vi "Get Filter Data.vi"(8 "error in (no error)":errorcluster, 11 "Filter XML Ref":refnum<k20>) -> (0 "error out":errorcluster, 1 "Parameters":T1[](array[typedef]) {"Base Word" format="%04d"; "Address" format="%04x"; "Mask" format="%04x"; "Value" format="%016x"}, 2 "Filter Configuration":T3, 3 "Name":string)   [LabVIEW 2016]
doc: "Retrieves all the Bus Monitor Filter Parameters and configuration from the Filter XML node. Each BMChannel should have a unique name. Each Filter should also have a unique name."
uses:
  <vilib>/xml/NI_XML.lvlib
  Frames & Messages/TypeDefs/Command Type.ctl
  BCI-1553 API.lvlib
  Filters/TypeDefs/Filter Configuration.ctl
  1553 SubComponent/TypeDefs/Scaling Information.ctl
  1553 SubComponent/1553 SubComponent.lvclass
  1553 SubComponent/TypeDefs/Parameter Table Data.ctl
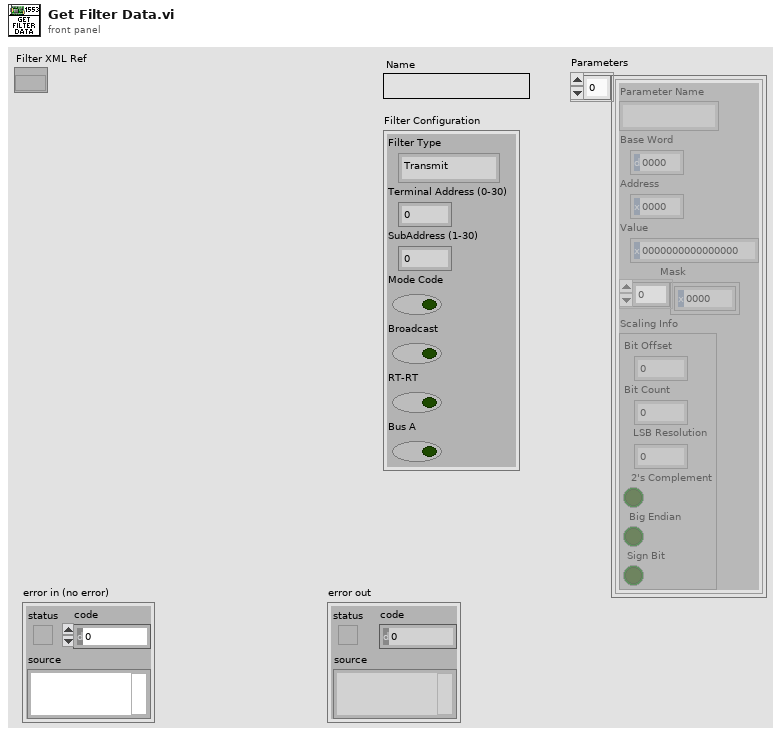
[diagram p1: front panel]
types:
  T1 = typedef "BCI-1553 API.lvlib/1553 SubComponent.lvclass/Parameter Table Data.ctl" = cluster{"Parameter Name":string, "Base Word":u16, "Address":u16, "Value":u64, "Mask":u16[], "Scaling Info":T2}
  T2 = typedef "BCI-1553 API.lvlib/1553 SubComponent.lvclass/Scaling Information.ctl" = cluster{"Bit Offset":i32, "Bit Count":i32, "LSB Resolution":dbl, "2's Complement":bool, "Big Endian":bool, "Sign Bit":bool}
  T3 = typedef "BCI-1553 API.lvlib/Filter Configuration.ctl" = cluster{"Filter Type":T4, "Terminal Address (0-30)":u16, "SubAddress (1-30)":u16, "Mode Code":bool, "Broadcast":bool, "RT-RT":bool, "Bus A":bool}
  T4 = typedef "BCI-1553 API.lvlib/Command Type.ctl" = enum16{"Transmit", "Receive"}
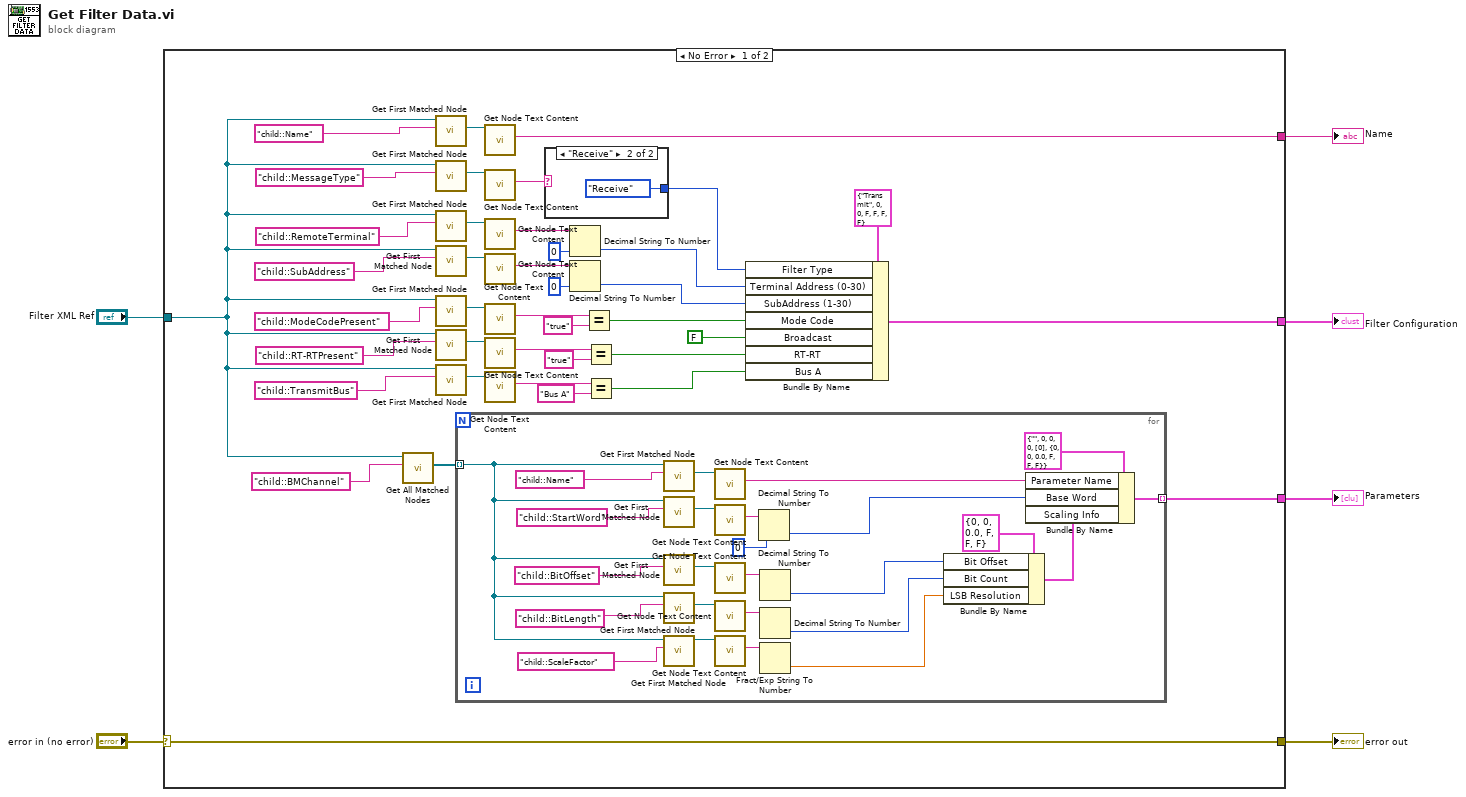
[diagram p0: block diagram]
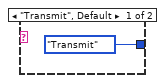
[diagram p2: hidden frame]
diagram:
  n1 = case shown="No Error" "error in (no error)" {
    selector: "error in (no error)" -> [w7 w74]
    tunnel: [w46 _] -> w6
    tunnel: "Filter XML Ref" -> [w45 _]
    tunnel: [w42 _] -> w4
    tunnel: [w41 _] -> w3
    tunnel: [w7 w74] -> w1
    frame No Error {
      n2 = call <vilib>:"Get All Matched Nodes.vi"("XPath expression"="child::BMChannel", "node in"=w45) -> ("node result array"=w40:refnum<k20>[])  [unwired: 7 in, 2 out]
      n3 = call <vilib>:"Get First Matched Node.vi"("XPath expression"="child::Name", "node in"=w45) -> ("node result"=w44:refnum<k20>)  [unwired: 7 in, 2 out]
      n4 = call <vilib>:"Get First Matched Node.vi"("XPath expression"="child::MessageType", "node in"=w45) -> ("node result"=w29:refnum<k20>)  [unwired: 7 in, 2 out]
      n5 = call <vilib>:"Get First Matched Node.vi"("XPath expression"="child::RemoteTerminal", "node in"=w45) -> ("node result"=w23:refnum<k20>)  [unwired: 7 in, 2 out]
      n6 = call <vilib>:"Get First Matched Node.vi"("XPath expression"="child::SubAddress", "node in"=w45) -> ("node result"=w24:refnum<k20>)  [unwired: 7 in, 2 out]
      n7 = call <vilib>:"Get First Matched Node.vi"("XPath expression"="child::ModeCodePresent", "node in"=w45) -> ("node result"=w25:refnum<k20>)  [unwired: 7 in, 2 out]
      n8 = call <vilib>:"Get First Matched Node.vi"("XPath expression"="child::RT-RTPresent", "node in"=w45) -> ("node result"=w26:refnum<k20>)  [unwired: 7 in, 2 out]
      n9 = call <vilib>:"Get First Matched Node.vi"("XPath expression"="child::TransmitBus", "node in"=w45) -> ("node result"=w27:refnum<k20>)  [unwired: 7 in, 2 out]
      n10 = for {
        tunnel: w40 -> [w57] mode=indexing
        tunnel: [w51] -> w41 mode=indexing
        n11 = call <vilib>:"Get First Matched Node.vi"("XPath expression"="child::Name", "node in"=w57) -> ("node result"=w61:refnum<k20>)  [unwired: 7 in, 2 out]
        n12 = call <vilib>:"Get First Matched Node.vi"("XPath expression"="child::StartWord", "node in"=w57) -> ("node result"=w60:refnum<k20>)  [unwired: 7 in, 2 out]
        n13 = call <vilib>:"Get First Matched Node.vi"("XPath expression"="child::BitOffset", "node in"=w57) -> ("node result"=w68:refnum<k20>)  [unwired: 7 in, 2 out]
        n14 = call <vilib>:"Get First Matched Node.vi"("XPath expression"="child::BitLength", "node in"=w57) -> ("node result"=w69:refnum<k20>)  [unwired: 7 in, 2 out]
        n15 = call <vilib>:"Get First Matched Node.vi"("XPath expression"="child::ScaleFactor", "node in"=w57) -> ("node out"=w65:refnum<k20>)  [unwired: 7 in, 2 out]
        n16 = call <vilib>:"Get Node Text Content.vi"("node in"=w61) -> ("node text"=w55:string)  [unwired: 8 in, 2 out]
        n17 = call <vilib>:"Get Node Text Content.vi"("node in"=w60) -> ("node text"=w58:string)  [unwired: 8 in, 2 out]
        n18 = call <vilib>:"Get Node Text Content.vi"("node in"=w68) -> ("node text"=w70:string)  [unwired: 8 in, 2 out]
        n19 = call <vilib>:"Get Node Text Content.vi"("node in"=w69) -> ("node text"=w71:string)  [unwired: 8 in, 2 out]
        n20 = call <vilib>:"Get Node Text Content.vi"("node in"=w65) -> ("node text"=w63:string)  [unwired: 8 in, 2 out]
        n21 = Decimal String To Number(string=w58, default (0L)=u16 0 ("default (0 I32)")) -> (number=w47:u16)  [unwired: 1 in, 1 out]
        n22 = Decimal String To Number(string=w70) -> (number=w50:i32)  [unwired: 2 in, 1 out]
        n23 = Decimal String To Number(string=w71) -> (number=w49:i32)  [unwired: 2 in, 1 out]
        n24 = Fract/Exp String To Number(string=w63) -> (number=w53:dbl)  [unwired: 3 in, 1 out]
        n25 = Bundle By Name(cluster=T2 {"Bit Offset"=0, "Bit Count"=0, "LSB Resolution"=0.0, "2's Complement"=FALSE, "Big Endian"=FALSE, "Sign Bit"=FALSE} ("Scaling Info"), "Bit Offset"=w50, "Bit Count"=w49, "LSB Resolution"=w53) -> (w52:T2)
        n26 = Bundle By Name(cluster=T1 {"Parameter Name"="", "Base Word"=0, "Address"=0, "Value"=0, "Mask"=[0], "Scaling Info"={"Bit Offset"=0, "Bit Count"=0, "LSB Resolution"=0.0, "2's Complement"=FALSE, "Big Endian"=FALSE, "Sign Bit"=FALSE}} ("Parameter Table Data"), "Parameter Name"=w55, "Base Word"=w47, "Scaling Info"=w52) -> (w51:T1)
      }
      n27 = call <vilib>:"Get Node Text Content.vi"("node in"=w44) -> ("node text"=w46:string)  [unwired: 8 in, 2 out]
      n28 = call <vilib>:"Get Node Text Content.vi"("node in"=w29) -> ("node text"=w36:string)  [unwired: 8 in, 2 out]
      n29 = call <vilib>:"Get Node Text Content.vi"("node in"=w23) -> ("node text"=w37:string)  [unwired: 8 in, 2 out]
      n30 = call <vilib>:"Get Node Text Content.vi"("node in"=w24) -> ("node text"=w38:string)  [unwired: 8 in, 2 out]
      n31 = call <vilib>:"Get Node Text Content.vi"("node in"=w25) -> ("node text"=w20:string)  [unwired: 8 in, 2 out]
      n32 = call <vilib>:"Get Node Text Content.vi"("node in"=w26) -> ("node text"=w16:string)  [unwired: 8 in, 2 out]
      n33 = call <vilib>:"Get Node Text Content.vi"("node in"=w27) -> ("node text"=w13:string)  [unwired: 8 in, 2 out]
      n34 = case shown="\"Receive\"" w36 {
        tunnel: [Command_Type."Transmit" ("Filter Type") Command_Type."Receive" ("Filter Type")] -> w21
        frame "Transmit", Default {
        }
        frame "Receive" {
        }
      }
      n35 = Decimal String To Number(string=w37, default (0L)=u16 0 ("default (0 I32)")) -> (number=w9:u16)  [unwired: 1 in, 1 out]
      n36 = Decimal String To Number(string=w38, default (0L)=u16 0 ("default (0 I32)")) -> (number=w8:u16)  [unwired: 1 in, 1 out]
      n37 = Equal?(x=w20, y="true") -> (x = y?=w18:bool)
      n38 = Equal?(x=w16, y="true") -> (x = y?=w15:bool)
      n39 = Equal?(x=w13, y="Bus A") -> (x = y?=w12:bool)
      n40 = Bundle By Name(cluster=T3 {"Filter Type"=enum."Transmit", "Terminal Address (0-30)"=0, "SubAddress (1-30)"=0, "Mode Code"=FALSE, "Broadcast"=FALSE, "RT-RT"=FALSE, "Bus A"=FALSE} ("Filter Configuration"), "Filter Type"=w21, "Terminal Address (0-30)"=w9, "SubAddress (1-30)"=w8, "Mode Code"=w18, "Broadcast"=FALSE, "RT-RT"=w15, "Bus A"=w12) -> (w42:T3)
    }
    frame Error {
    }
  }
  "Name" <- w6
  "Filter Configuration" <- w4
  "Parameters" <- w3
  "error out" <- w1
